vi "Offset_Static_Dynamic_Test.vi"(0 "Semiconductor Module Context":T7, 1 "Pins Force":T2[](array[typedef]), 2 "Pins Meas":T2[](array[typedef]), 3 "DCPower_Parameters":T1={"Output"=enum."DC Voltage", "Current_range"=0.0, "Current"=0.0, "Voltage_range"=0.0, "Voltage"=0.0, "Aperture_time"=0.0, "Source Delay"=0.0, "Sense"=1008} {"Source Delay" format="%.6p"; "Sense" items=["Local"=1008, "Remote"=1009]; "Aperture_time" format="%.6p"; "Current_range" format="%.6p"; "Current" format="%.6p"; "Voltage_range" format="%.6p"; "Voltage" format="%.6p"}, 4 "FGEN_Parameters":T3 {"Trigger Mode" items=["Single", "Continuous", "Stepped", "Burst"]}, 5 "SCOPE_Parameters":T5={"min sample rate"=20000000.0, "min record length"=1000, "reference position"=5.0, "input impedance"=0, "maximum input frequency"=0.0, "vertical coupling"=1, "vertical range"=10.0, "vertical offset"=0.0, "NumRecords"=0} {"maximum input frequency" format="%.2f"; "input impedance" items=["1 mega ohm"=0, "50 ohms"=2]; "vertical offset" format="%.4f"; "vertical range" format="%.2f"; "vertical coupling" items=["AC", "DC", "Ground"]; "reference position" format="%#_13g"; "min sample rate" format="%^.2e"}, 7 "Source Type":enum16{"Static", "Dynamic"}(ring)) -> (19 "error out":errorcluster)   [LabVIEW 2023, in "Offset.lvlib"]
doc: "Configures SMU/AWG and start generating; if using SMU it also measures back the voltage applied.\nThe SCOPE acquires N channels and averages the samples of each channel.\nThe Offset is computed by dividing the average value with the applied voltage or Vrms of Sine wave when using AWG"
uses:
  Offset.lvlib
  <vilib>/NI_TestStand_SemiconductorModule/NI_TestStand_Semiconductor_Module.lvlibp/PinMap/General/SemiconductorModuleContext.ctl
  <vilib>/NI_TestStand_SemiconductorModule/NI_TestStand_Semiconductor_Module.lvlibp/PinMap/TagProvider/TSM_Pin.ctl
  ResourceHandling/TypeDefs/RH_SCOPE_Parameters.ctl
  <instrlib>/niScope/Controls/niScope vertical coupling.ctl
  ResourceHandling/TypeDefs/RH_FGEN_Parameters.ctl
  <instrlib>/niFgen/niFgen.llb/niFgen Trigger Mode.ctl
  ResourceHandling/TypeDefs/RH_DCPower_Parameters.ctl
  <vilib>/Analysis/baseanly.llb/Mean (DBL).vi
  <vilib>/NI_TestStand_SemiconductorModule/NI_TestStand_Semiconductor_Module.lvlibp/PinMap/PinQueryContext/MultiplePinSingleSessionQueryContext/MultiplePinSingleSessionQueryContext.lvclass
  C:/Program Files/National Instruments/LabVIEW 2023/vi.lib/NI_TestStand_SemiconductorModule/NI_TestStand_Semiconductor_Module.lvlibp/PinMap/PinQueryContext/PinQueryContext.lvclass
  <vilib>/NI_TestStand_SemiconductorModule/NI_TestStand_Semiconductor_Module.lvlibp/PinMap/DC Power/PinsToNIDCPowerSessions.vi
  <vilib>/NI_TestStand_SemiconductorModule/NI_TestStand_Semiconductor_Module.lvlibp/PinMap/FGEN/PinToNIFGenSession.vi
  <vilib>/NI_TestStand_SemiconductorModule/NI_TestStand_Semiconductor_Module.lvlibp/PinMap/Scope/PinsToNISCOPESession.vi
  <instrlib>/niScope/Acquire/Fetch/niScope Multi Fetch WDT.vi
  <vilib>/NI_TestStand_SemiconductorModule/NI_TestStand_Semiconductor_Module.lvlibp/PinMap/General/Publish/PublishDataDouble1D.vi
  ResourceHandling/ResourceHandling.lvlib
  <vilib>/NI_TestStand_SemiconductorModule/NI_TestStand_Semiconductor_Module.lvlibp
  <vilib>/Analysis/NI_AALBase.lvlib
  C:/Program Files/National Instruments/LabVIEW 2023/vi.lib/NI_TestStand_SemiconductorModule/NI_TestStand_Semiconductor_Module.lvlibp/PinMap/PinQueryContext/MultiplePinSingleSessionQueryContext/MultiplePinSingleSessionQueryContext.lvclass
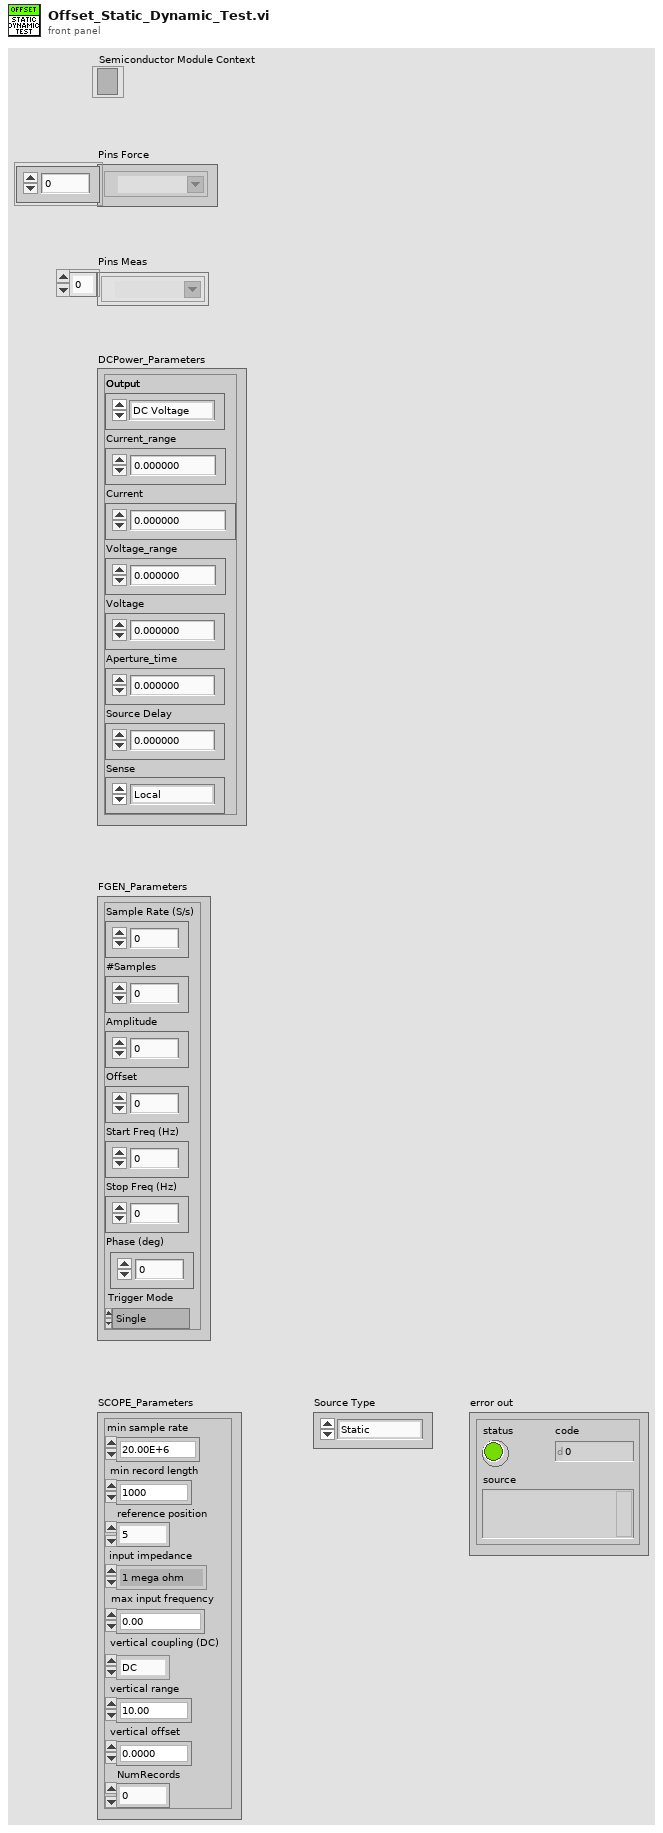
[diagram p1: front panel]
types:
  T1 = typedef "ResourceHandling.lvlib/RH_DCPower_Parameters.ctl" = cluster{"Output":enum16{"DC Voltage", "DC Current"}, "Current_range":dbl, "Current":dbl, "Voltage_range":dbl, "Voltage":dbl, "Aperture_time":dbl, "Source Delay":dbl, "Sense":i32}
  T2 = typedef "NI_TestStand_Semiconductor_Module.lvlibp/TSM_Pin.ctl" = tag
  T3 = typedef "ResourceHandling.lvlib/RH_FGEN_Parameters.ctl" = cluster{"Sample Rate (S/s)":dbl, "#Samples":i32, "Amplitude":dbl, "Offset":dbl, "Start Freq (Hz)":dbl, "Stop Freq (Hz)":dbl, "Phase (deg)":dbl, "Trigger Mode":T4}
  T4 = typedef "niFgen Trigger Mode.ctl" = i32
  T5 = typedef "ResourceHandling.lvlib/RH_SCOPE_Parameters.ctl" = cluster{"min sample rate":dbl, "min record length":i32, "reference position":dbl, "input impedance":u32, "maximum input frequency":dbl, "vertical coupling":T6, "vertical range":dbl, "vertical offset":dbl, "NumRecords":i32}
  T6 = typedef "niScope vertical coupling.ctl" = i32
  T7 = typedef "NI_TestStand_Semiconductor_Module.lvlibp/SemiconductorModuleContext.ctl" = refnum<k7>
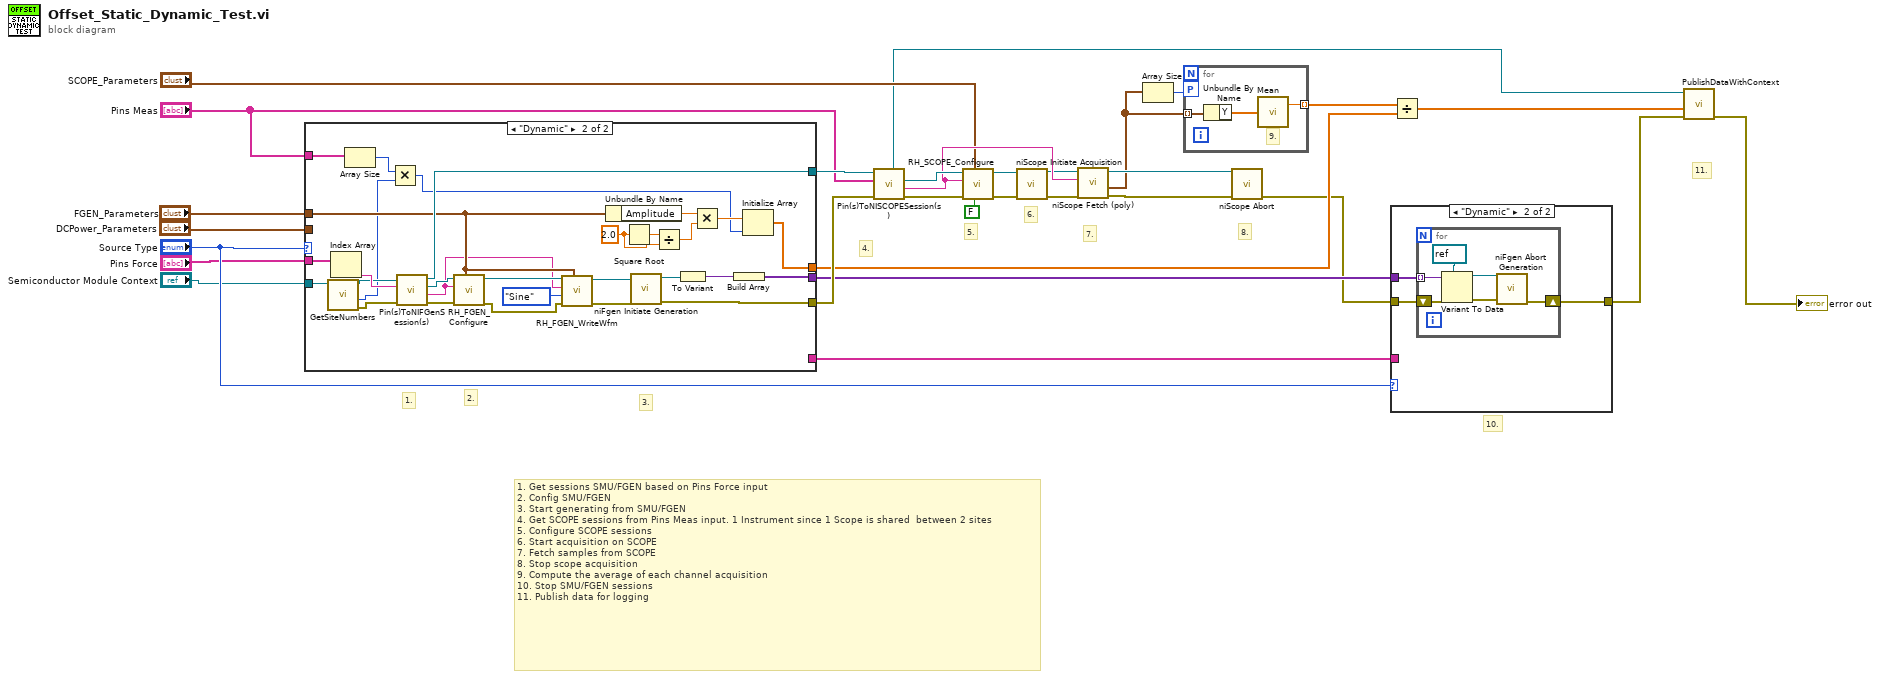
[diagram p0: block diagram]
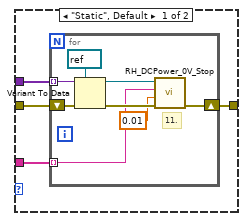
[diagram p2: hidden frame]
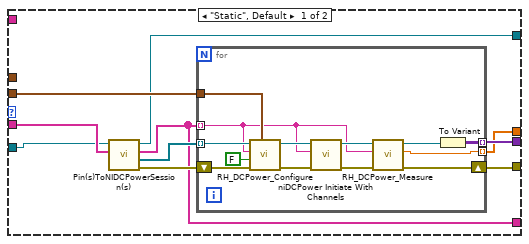
[diagram p3: hidden frame]
diagram:
  # "10."
  # "1."
  # "11."
  # "8."
  # "7."
  # "6."
  # "5."
  # "4."
  # "3."
  # "2."
  # "1. Get sessions SMU/FGEN based on Pins Force input\n2. Config SMU/FGEN\n3. Start generating from SMU/FGEN\n4. Get SCOPE sessions from Pins Meas input. 1 Instrument since 1 Scope is shared  between 2 sites\n5. Configure SCOPE sessions\n6. Start acquisition on SCOPE\n7. Fetch samples from SCOPE\n8. Stop scope acquisition\n9. Compute the average of each channel acquisition\n10. Stop SMU/FGEN sessions\n11. Publish data for logging"
  n1 = case shown="\"Dynamic\"" "Source Type" {
    tunnel: [w37 w80] -> w25
    tunnel: "Pins Force" -> [w32 w72]
    tunnel: "DCPower_Parameters" -> [w38 _]
    tunnel: [w36 w82] -> w29
    tunnel: [w35 w73] -> w24
    tunnel: "FGEN_Parameters" -> [_ w66]
    tunnel: [w34 w60] -> w22
    tunnel: [w33 _] -> w23
    tunnel: "Semiconductor Module Context" -> [w31 w59]
    tunnel: "Pins Meas" -> [_ w62]
    frame "Static", Default {
      n2 = call-poly <vilib>:"Pin(s)ToNIDCPowerSession(s).vi"("Pins"=w32, "Semiconductor Module Context"=w31) -> ("error out"=w40:errorcluster, "Instrument Sessions"=w39:refnum<k15>[], "Channel Strings"=w33:string[], "Semiconductor Module Context Out"=w36:T7)  [unwired: 5 in, 1 out]
      n3 = for {
        shift-right: [w42] -> w37
        shift-left: w40 -> [w53]
        tunnel: w39 -> [w51] mode=indexing
        tunnel: w33 -> [w44] mode=indexing
        tunnel: w38 -> [w50]
        tunnel: [w47] -> w35 mode=indexing
        tunnel: [w41] -> w34 mode=indexing
        n4 = call "RH_DCPower_Configure.vi"("DCPower_Parameters"=w50, "error in (no error)"=w53, "trigger out?"=FALSE, "channel name"=w44, "DCPower Session In"=w51) -> ("error out"=w49:errorcluster, "DCPower Session Out"=w48:refnum<k15>)  [unwired: 5 in]
        n5 = call <instrlib>:"niDCPower Initiate With Channels.vi"("error in (no error)"=w49, "channel name"=w44, "instrument handle"=w48) -> ("error out"=w46:errorcluster, "instrument handle out"=w45:refnum<k15>)  [unwired: 7 in]
        n6 = call "RH_DCPower_Measure.vi"("error in (no error)"=w46, "channel name"=w44, "DCPower Session In"=w45) -> ("error out"=w42:errorcluster, "Voltage"=w41:dbl, "DCPower Session Out"=w43:refnum<k15>)  [unwired: 5 in, 1 out]
        n7 = To Variant(anything=w43) -> (Variant=w47:variant)
      }
    }
    frame "Dynamic" {
      w75 = 2.0 ("x")
      n8 = call <vilib>:"GetSiteNumbers.vi"("Semiconductor Module Context"=w59) -> ("error out"=w57:errorcluster, "Number Of Sites"=w56:i32, "Semiconductor Module Context Out"=w58:T7)  [unwired: 7 in, 1 out]
      n9 = Index Array(array=w72) -> (element=w71:T2)  [unwired: 1 in]
      n10 = Array Size(array=w62) -> (size(s)=w55:i32)
      n11 = Multiply(x=w55, y=w56) -> (x*y=w54:i32)
      n12 = call-poly <vilib>:"Pin(s)ToNIFGenSession(s).vi"("error in (no error)"=w57, "Pin"=w71, "Semiconductor Module Context"=w58) -> ("error out"=w70:errorcluster, "Channel List"=w63:string, "Instrument Session"=w69:refnum<k15>, "Semiconductor Module Context Out"=w82:T7)  [unwired: 4 in, 1 out]
      n13 = call "RH_FGEN_Configure.vi"("FGEN Parameters"=w66, "error in"=w70, "Channel Name"=w63, "FGEN Session In"=w69) -> ("error out"=w65:errorcluster, "FGEN Session Out"=w68:refnum<k15>)  [unwired: 6 in]
      n14 = call "RH_FGEN_WriteWfm.vi"("FGEN Parameters"=w66, "error IO"=w65, "Wfm Type"=enum16{"Chirp", "MultiSine", "Sine"}."Sine", "Channel Name"=w63, "FGEN Session In"=w68) -> ("error out"=w64:errorcluster, "FGEN Session Out"=w67:refnum<k15>)  [unwired: 5 in]
      n15 = Unbundle By Name(w66) -> ("Amplitude"=w77:dbl)
      n16 = Square Root(x=w75) -> (sqrt(x)=w76:dbl)
      n17 = call <instrlib>:"niFgen Initiate Generation.vi"("error in (no error)"=w64, "Instrument Handle"=w67) -> ("error out"=w80:errorcluster, "Instrument Handle Out"=w78:refnum<k15>)  [unwired: 8 in]
      n18 = Divide(x=w76, y=w75) -> (x/y=w74:dbl)
      n19 = To Variant(anything=w78) -> (Variant=w81:variant)
      n20 = Multiply(x=w77, y=w74) -> (x*y=w61:dbl)
      n21 = Build Array(w81) -> (w73:variant[])
      n22 = Initialize Array(w61, w54) -> (w60:dbl[])
    }
  }
  n23 = call-poly <vilib>:"Pin(s)ToNISCOPESession(s).vi"("error in (no error)"=w25, "Pins"="Pins Meas", "Semiconductor Module Context"=w29) -> ("error out"=w26:errorcluster, "Channel List"=w27:string, "Instrument Session"=w28:refnum<k15>, "Pin Query Context"=w8:refnum<class "MultiplePinSingleSessionQueryContext.lvclass">)  [unwired: 4 in, 1 out]
  n24 = call "RH_SCOPE_Configure.vi"("Digital Trigger?"=FALSE, "SCOPE Global Parameters"="SCOPE_Parameters", "error in"=w26, "channels"=w27, "SCOPE Session In"=w28) -> ("error out"=w17:errorcluster, "SCOPE Session Out"=w18:refnum<k15>)  [unwired: 5 in]
  n25 = call <instrlib>:"niScope Initiate Acquisition.vi"("instrument handle"=w18, "error in"=w17) -> ("instrument handle out"=w16:refnum<k15>, "error out"=w15:errorcluster)  [unwired: 12 in]
  n26 = call-poly <instrlib>:"niScope Fetch (poly).vi"("error in"=w15, "channels"=w27, "instrument handle"=w16) -> ("error out"=w13:errorcluster, "wfm"=w2:waveform(dbl)[], "instrument handle out"=w14:refnum<k15>)  [unwired: 5 in, 1 out]
  n27 = Array Size(array=w2) -> (size(s)=w3:i32)
  n28 = for {
    tunnel: w2 -> [w84] mode=indexing
    tunnel: [w85] -> w10 mode=indexing
    workers-P: w3 -> [_]
    # "9."
    n29 = Unbundle By Name(w84) -> ("Y"=w83:dbl[])
    n30 = call-poly <vilib>:"Mean.vi"("X"=w83) -> ("mean"=w85:dbl)  [unwired: 1 out]
  }
  n31 = call <instrlib>:"niScope Abort.vi"("instrument handle"=w14, "error in"=w13) -> ("error out"=w7:errorcluster)  [unwired: 12 in, 1 out]
  n32 = case shown="\"Dynamic\"" "Source Type" {
    tunnel: w24 -> [w89 w100]
    tunnel: w7 -> [w88 w99]
    tunnel: w23 -> [w87 _]
    tunnel: [w86 w98] -> w6
    frame "Static", Default {
      n33 = for {
        tunnel: w89 -> [w97] mode=indexing
        tunnel: w87 -> [w92] mode=indexing
        shift-right: [w90] -> w86
        shift-left: w88 -> [w93]
        # "11."
        n34 = Variant To Data(error in=w93, type=refnum<k15> refnum ("DCPower Session In"), Variant=w97) -> (data=w95:refnum<k15>, error out=w94:errorcluster)
        n35 = call "RH_DCPower_0V_Stop.vi"("error in (no error)"=w94, "Settling (s)"=0.01, "Channel List"=w92, "DCPower Session In"=w95) -> ("error out"=w90:errorcluster)  [unwired: 6 in, 1 out]
      }
    }
    frame "Dynamic" {
      n36 = for {
        tunnel: w100 -> [w106] mode=indexing
        shift-right: [w101] -> w98
        shift-left: w99 -> [w105]
        n37 = Variant To Data(error in=w105, type=refnum<k15> refnum ("Instrument Handle"), Variant=w106) -> (data=w103:refnum<k15>, error out=w102:errorcluster)
        n38 = call <instrlib>:"niFgen Abort Generation.vi"("error in (no error)"=w102, "Instrument Handle"=w103) -> ("error out"=w101:errorcluster)  [unwired: 8 in, 1 out]
      }
    }
  }
  n39 = Divide(x=w10, y=w22) -> (x/y=w9:dbl[])
  n40 = call-poly <vilib>:"PublishDataWithContext.vi"("error in (no error)"=w6, "Data In"=w9, "Pin Query Context"=w8) -> ("error out"=→"error out":errorcluster)  [unwired: 7 in, 1 out]
